vi "Test Lidar.vi"() -> ()   [LabVIEW 2017]
panel:
  out "Loop Time":u32
  out "XY Graph":cluster{dbl[], dbl[]}(graph)
  in  "stop":bool
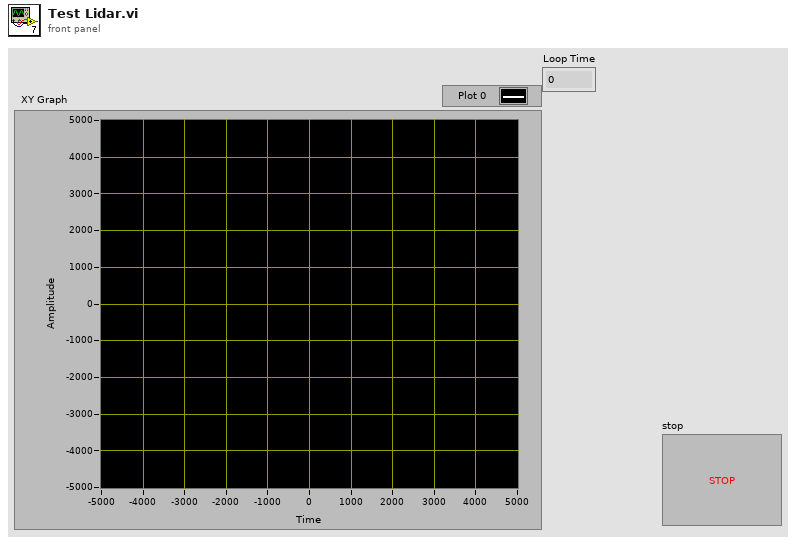
[diagram p1: front panel]
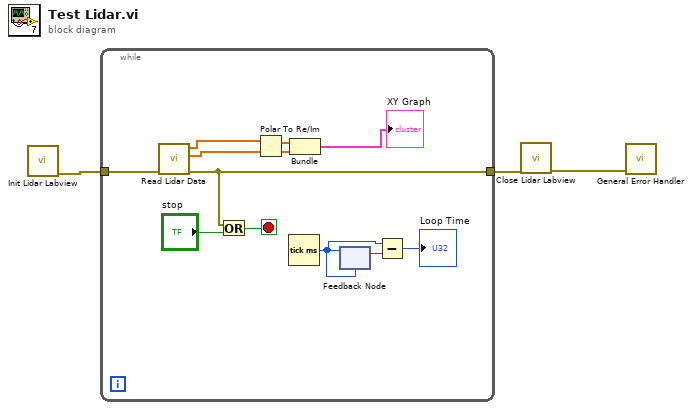
[diagram p0: block diagram]
diagram:
  n1 = call "Init Lidar Labview.vi"() -> ("error out"=w3:errorcluster)  [unwired: 11 in]
  n2 = while {
    tunnel: w3 -> [w15]
    tunnel: [w13] -> w2
    stop <- w14 stop-if-true
    n3 = call "Read Lidar Data.vi"("error in (no error)"=w15) -> ("error out"=w13:errorcluster, "Direction"=w4:dbl[], "Magnitude"=w5:dbl[])  [unwired: 8 in]
    n4 = Or(x=w13, y="stop") -> (x .or. y?=w14:bool)
    n5 = Polar To Re/Im(2:w4, 3:w5) -> (0:w10:dbl[], 1:w11:dbl[])
    n6 = Tick Count (ms)() -> (millisecond timer value=w8:u32)
    n7 = Bundle(w11, w10) -> (→"XY Graph":cluster{dbl[], dbl[]})  [unwired: 1 in]
    n8 = feedback-in #1(w8) -> ()
    n9 = feedback #1(w8) -> (w7:u32)
    n10 = Subtract(x=w8, y=w7) -> (x-y=→"Loop Time":u32)
  }
  n11 = call "Close Lidar Labview.vi"("error in (no error)"=w2) -> ("error out"=w1:errorcluster)  [unwired: 10 in]
  n12 = call <vilib>:"General Error Handler.vi"("error in (no error)"=w1) -> ()  [unwired: 10 in, 5 out]
